vi "DB_WriteInGen1.vi"(8 "error in (no error)":errorcluster, 9 "Equipo_Medicion":T2, 10 "PM_out":T1={"Equipo_Medicion"={"ID_EQUIPO"=0, "IP_EQUIPO"="", "NOMBRE_EQUIPO"="", "ESTADO_EQUIPO"="", "DESCRIPCION"="", "ID_MEDICION"=0, "ESTADO_MEDICION"="", "TIEMPO_MEDICION"="12-02-2019 18:41"}, "VIF_cluster"={"VL_VL"={"V1_V2"=0.0, "V2_V3"=0.0, "V3_V1"=0.0, "Avg_VL_VL"=0.0}, "IL_IL"={"I1"=0.0, "I2"=0.0, "I3"=0.0, "Avg_Amps"=0.0}, "Frecuency"=0.0, "Avg_Frecuency"=0.0}, "Power_cluster"={"Real Power (kW)"={"L1_kW"=0.0, "L2_kW"=0.0, "L3_kW"=0.0, "Total_kW"=0.0}, "Reactive Power (kVAR)"={"L1_kVAR"=0.0, "L2_kVAR"=0.0, "L3_kVAR"=0.0, "Total_kVAR"=0.0}, "Aparent Power (kVA)"={"L1_kVA"=0.0, "L2_kVA"=0.0, "L3_kVA"=0.0, "Total_kVA"=0.0}, "Power Factor (%)"={"L1_PF"=0.0, "L2_PF"=0.0, "L3_PF"=0.0, "Total_PF"=0.0}}, "THD_cluster"={"V_THD"={"V1_V2_THD"=0.0, "V2_V3_THD"=0.0, "V3_V1_THD"=0.0, "Avg_V_V_THD"=0.0}, "I_THD"={"I1_THD"=0.0, "I2_THD"=0.0, "I3_THD"=0.0, "I4_THD"=0.0, "Avg_I_THD"=0.0}}, "Polar_cluster"={"V_polar"={"V1_ang"=0.0, "V1_mag"=0.0, "V2_ang"=0.0, "V2_mag"=0.0, "V3_ang"=0.0, "V3_mag"=0.0}, "I_polar"={"I1_ang"=0.0, "I1_mag"=0.0, "I2_ang"=0.0, "I2_mag"=0.0, "I3_ang"=0.0, "I3_mag"=0.0}}}, 11 "DB in":T7) -> (0 "error out":errorcluster, 3 "closeDB":T7[](array[typedef]))   [LabVIEW 2018]
uses:
  <vilib>/addons/database/Connection.llb/Conn ObjectReference.ctl
  Controls/Equipos_Medicion_cluster.ctl
  Controls/Cluster_Data.ctl
  Controls/VIF_cluster.ctl
  Controls/Power_cluster.ctl
  Controls/THD_cluster.ctl
  Controls/Polar_cluster.ctl
  <vilib>/addons/database/NI_Database_API.lvlib
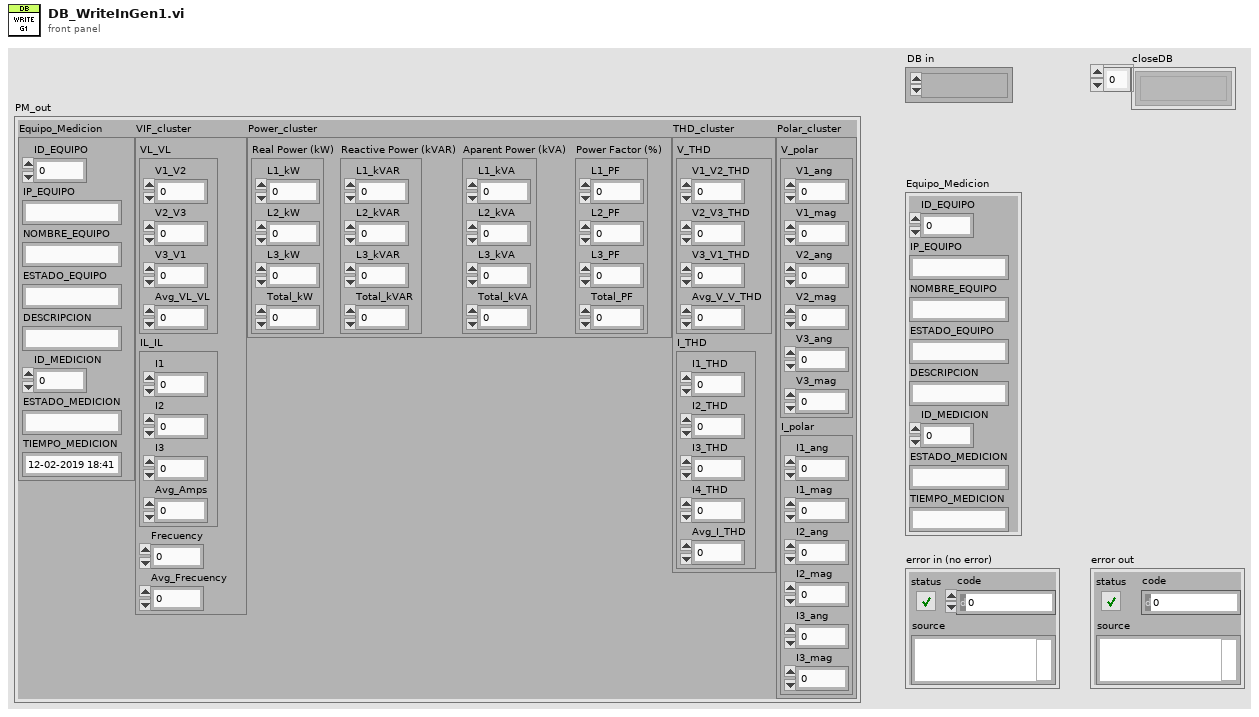
[diagram p1: front panel]
types:
  T1 = typedef "Cluster_Data.ctl" = cluster{"Equipo_Medicion":T2, "VIF_cluster":T3, "Power_cluster":T4, "THD_cluster":T5, "Polar_cluster":T6}
  T2 = typedef "Equipos_Medicion_cluster.ctl" = cluster{"ID_EQUIPO":i32, "IP_EQUIPO":string, "NOMBRE_EQUIPO":string, "ESTADO_EQUIPO":string, "DESCRIPCION":string, "ID_MEDICION":i32, "ESTADO_MEDICION":string, "TIEMPO_MEDICION":string}
  T3 = typedef "VIF_cluster.ctl" = cluster{"VL_VL":cluster{"V1_V2":sgl, "V2_V3":sgl, "V3_V1":sgl, "Avg_VL_VL":sgl}, "IL_IL":cluster{"I1":sgl, "I2":sgl, "I3":sgl, "Avg_Amps":sgl}, "Frecuency":sgl, "Avg_Frecuency":sgl}
  T4 = typedef "Power_cluster.ctl" = cluster{"Real Power (kW)":cluster{"L1_kW":sgl, "L2_kW":sgl, "L3_kW":sgl, "Total_kW":sgl}, "Reactive Power (kVAR)":cluster{"L1_kVAR":sgl, "L2_kVAR":sgl, "L3_kVAR":sgl, "Total_kVAR":sgl}, "Aparent Power (kVA)":cluster{"L1_kVA":sgl, "L2_kVA":sgl, "L3_kVA":sgl, "Total_kVA":sgl}, "Power Factor (%)":cluster{"L1_PF":sgl, "L2_PF":sgl, "L3_PF":sgl, "Total_PF":sgl}}
  T5 = typedef "THD_cluster.ctl" = cluster{"V_THD":cluster{"V1_V2_THD":sgl, "V2_V3_THD":sgl, "V3_V1_THD":sgl, "Avg_V_V_THD":sgl}, "I_THD":cluster{"I1_THD":sgl, "I2_THD":sgl, "I3_THD":sgl, "I4_THD":sgl, "Avg_I_THD":sgl}}
  T6 = typedef "Polar_cluster.ctl" = cluster{"V_polar":cluster{"V1_ang":sgl, "V1_mag":sgl, "V2_ang":sgl, "V2_mag":sgl, "V3_ang":sgl, "V3_mag":sgl}, "I_polar":cluster{"I1_ang":sgl, "I1_mag":sgl, "I2_ang":sgl, "I2_mag":sgl, "I3_ang":sgl, "I3_mag":sgl}}
  T7 = typedef "NI_Database_API.lvlib/Conn ObjectReference.ctl" = refnum<k1>
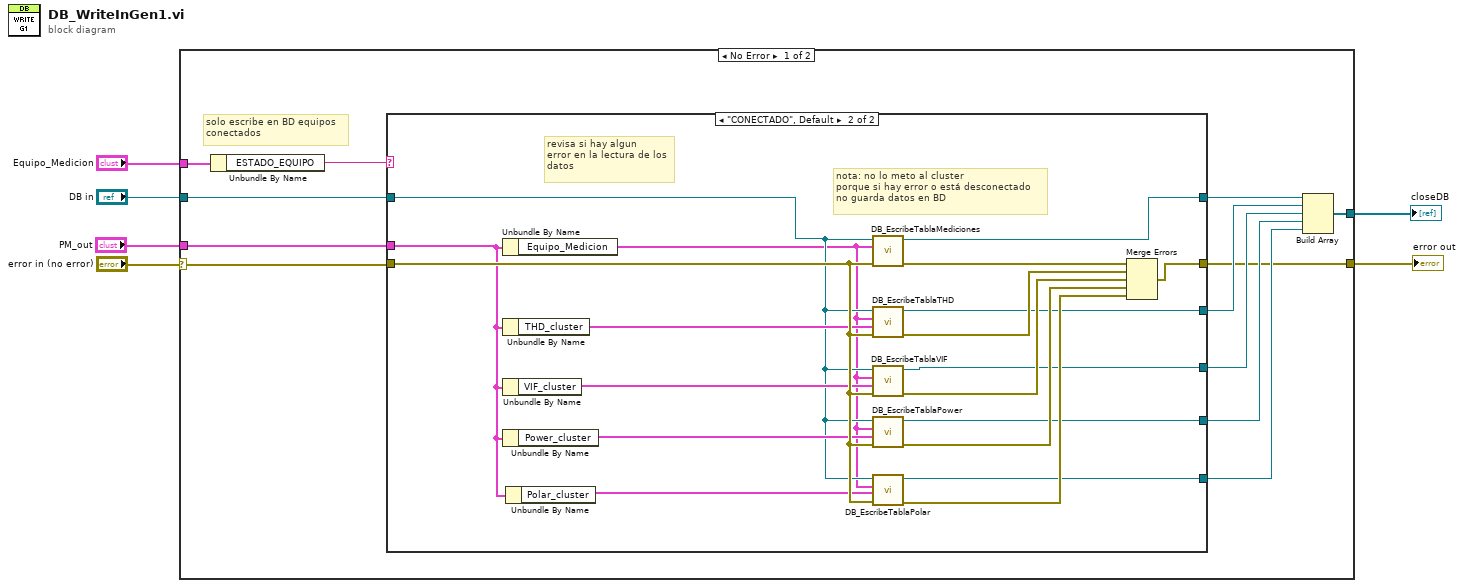
[diagram p0: block diagram]
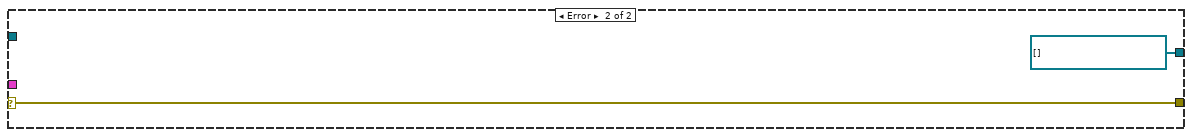
[diagram p3: hidden frame]
diagram:
  n1 = case shown="No Error" "error in (no error)" {
    selector: "error in (no error)" -> [w8 w40]
    tunnel: [w18 w41] -> w6
    tunnel: "Equipo_Medicion" -> [w12 _]
    tunnel: "DB in" -> [w11 _]
    tunnel: [w10 w40] -> w3
    tunnel: "PM_out" -> [w9 _]
    frame No Error {
      # "solo escribe en BD equipos\nconectados"
      n2 = Unbundle By Name(w12) -> ("ESTADO_EQUIPO"=w7:string)
      n3 = case shown="\"CONECTADO\", Default" w7 {
        tunnel: w8 -> [w20 w39]
        tunnel: w11 -> [w19 w22]
        tunnel: [w20 w38] -> w10
        tunnel: [w19 w28] -> w13
        tunnel: [_ w27] -> w17
        tunnel: [_ w26] -> w16
        tunnel: [_ w25] -> w15
        tunnel: [_ w24] -> w14
        tunnel: w9 -> [_ w23]
        frame "DESCONECTADO" {
          # "Equipo está deconectado"
        }
        frame "CONECTADO", Default {
          # "nota: no lo meto al cluster\nporque si hay error o está desconectado\nno guarda datos en BD"
          # "revisa si hay algun \nerror en la lectura de los\ndatos"
          n4 = Unbundle By Name(w23) -> ("Equipo_Medicion"=w21:T2)
          n5 = Unbundle By Name(w23) -> ("THD_cluster"=w37:T5)
          n6 = Unbundle By Name(w23) -> ("VIF_cluster"=w36:T3)
          n7 = Unbundle By Name(w23) -> ("Power_cluster"=w35:T4)
          n8 = Unbundle By Name(w23) -> ("Polar_cluster"=w34:T6)
          n9 = call "DB_EscribeTablaMediciones.vi"("error in (no error)"=w39, "Equipo_Medicion in"=w21, "db in"=w22) -> ("error out"=w33:errorcluster, "db out"=w28:T7)  [unwired: 7 in]
          n10 = call "DB_EscribeTablaTHD.vi"("error in (no error)"=w39, "THD_cluster"=w37, "Equipo_Medicion"=w21, "db in"=w22) -> ("error out"=w32:errorcluster, "db out"=w24:T7)  [unwired: 6 in]
          n11 = call "DB_EscribeTablaVIF.vi"("error in (no error)"=w39, "VIF_cluster"=w36, "Equipo_Medicion"=w21, "db in"=w22) -> ("error out"=w31:errorcluster, "db out"=w25:T7)  [unwired: 6 in]
          n12 = call "DB_EscribeTablaPower.vi"("error in (no error)"=w39, "Power_cluster"=w35, "Equipo_Medicion"=w21, "db in"=w22) -> ("error out"=w30:errorcluster, "db out"=w26:T7)  [unwired: 6 in]
          n13 = call "DB_EscribeTablaPolar.vi"("error in (no error)"=w39, "Polar_cluster"=w34, "Equipo_Medicion"=w21, "db in"=w22) -> ("error out"=w29:errorcluster, "db out"=w27:T7)  [unwired: 6 in]
          n14 = Merge Errors(w33, w32, w31, w30, w29) -> (w38:errorcluster)
        }
      }
      n15 = Build Array(w13, w14, w15, w16, w17) -> (w18:T7[])
    }
    frame Error {
      w41 = T7[] [] items=["Connection"]
    }
  }
  "closeDB" <- w6
  "error out" <- w3
